vi "(SubVI) Setup a Sine Wave Configuration.vi"(6 "Amplitude (nm)":dbl, 7 "freq. (Hz)":dbl, 10 "Axis Enum":enum16{"x", "y", "z"}(ring), 11 "Current Commanded position (um)":dbl) -> (0 "error out":errorcluster)   [LabVIEW 2014]
panel:
  in  "Sine Parameters:":T1={"Xo (Start)"=0, "SIN_P Parameters"={"C"=200.0, "A"=10.0, "O"=0.0}, "N (Length)"=500, "Append? (&)"=FALSE} {"N (Length)" min=0 max=1000 step=1; "SIN_P Parameters"."O" format="%.6f"; "SIN_P Parameters"."A" format="%.6f"; "SIN_P Parameters"."C" format="%.6f"}
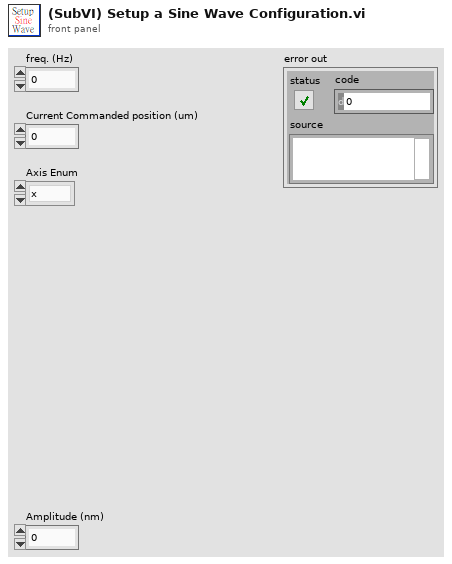
[diagram p1: front panel]
types:
  T1 = cluster{"Xo (Start)":i32, "SIN_P Parameters":cluster{"C":dbl, "A":dbl, "O":dbl}, "N (Length)":i32, "Append? (&)":bool}
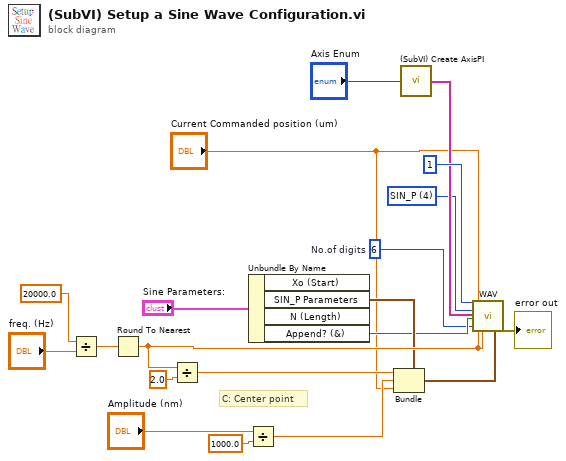
[diagram p0: block diagram]
diagram:
  w2 = i16 6  # No.of digits
  w3 = u16 4 items=["SIN", "POL", "TAN", "PNT", "SIN_P", "LIN", "RAMP"] ("Waveform")
  # "C: Center point"
  n1 = Divide(x=20000.0, y="freq. (Hz)") -> (x/y=w9:dbl)
  n2 = Round To Nearest(number=w9) -> (nearest integer value=w12:dbl)
  n3 = Divide(x=w12, y=2.0) -> (x/y=w14:dbl)
  n4 = Divide(x="Amplitude (nm)", y=1000.0) -> (x/y=w17:dbl)
  n5 = Unbundle By Name("Sine Parameters:") -> ("SIN_P Parameters"=w11:cluster{"C":dbl, "A":dbl, "O":dbl}, "Append? (&)"=w6:bool)  [unwired: 2 out]
  n6 = Bundle(cluster=w11, "C"=w14, "A"=w17, "O"="Current Commanded position (um)") -> (w18:cluster{"C":dbl, "A":dbl, "O":dbl})
  n7 = call "(SubVI) Create AxisPI.vi"("axis"="Axis Enum") -> ("Axis String Array"=w4:string[])  [unwired: 2 in, 2 out]
  n8 = call "WAV.vi"("System no."=1, "Waveform"=w3, "Affected axes"=w4, "Append? (&)"=w6, "No.of digits"=w2, "Xo"="Current Commanded position (um)", "N"=w12, "Segment length"=w12, "SIN_P Parameters"=w18) -> ("error out"=→"error out":errorcluster)  [unwired: 11 in, 7 out]
